vi "Pos_ImageIO.vi"(7 "Pos_ImageIO_commands":T2, 8 "Error In":errorcluster, 10 "Image File Path":path, 11 "ImageCluster IN":cluster{"Current Image":T1, "Saved Image":T1}) -> (0 "Error Out":errorcluster, 2 "Error!":bool, 3 "Saved Image OUT":T1)   [LabVIEW 2012]
uses:
  Pos_ImageIO_commands.ctl
  <vilib>/vision/Image Controls.llb/IMAQ Image.ctl
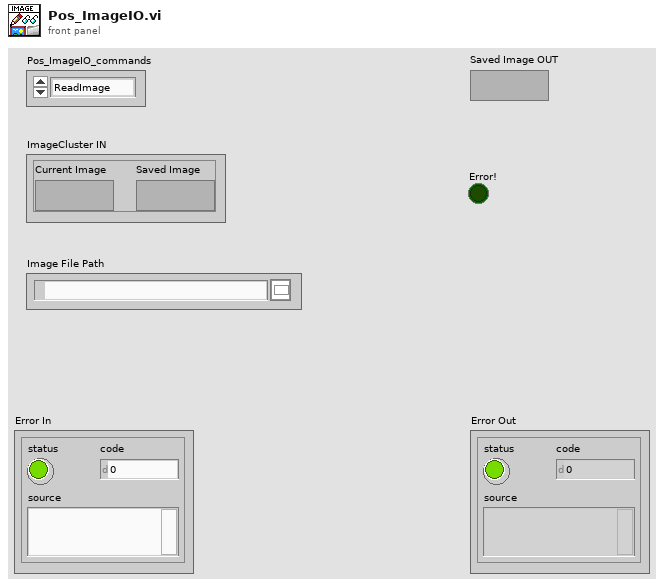
[diagram p1: front panel]
types:
  T1 = typedef "IMAQ Image.ctl" = refnum<image>
  T2 = typedef "Pos_ImageIO_commands.ctl" = enum16{"ReadImage", "WriteImage"}
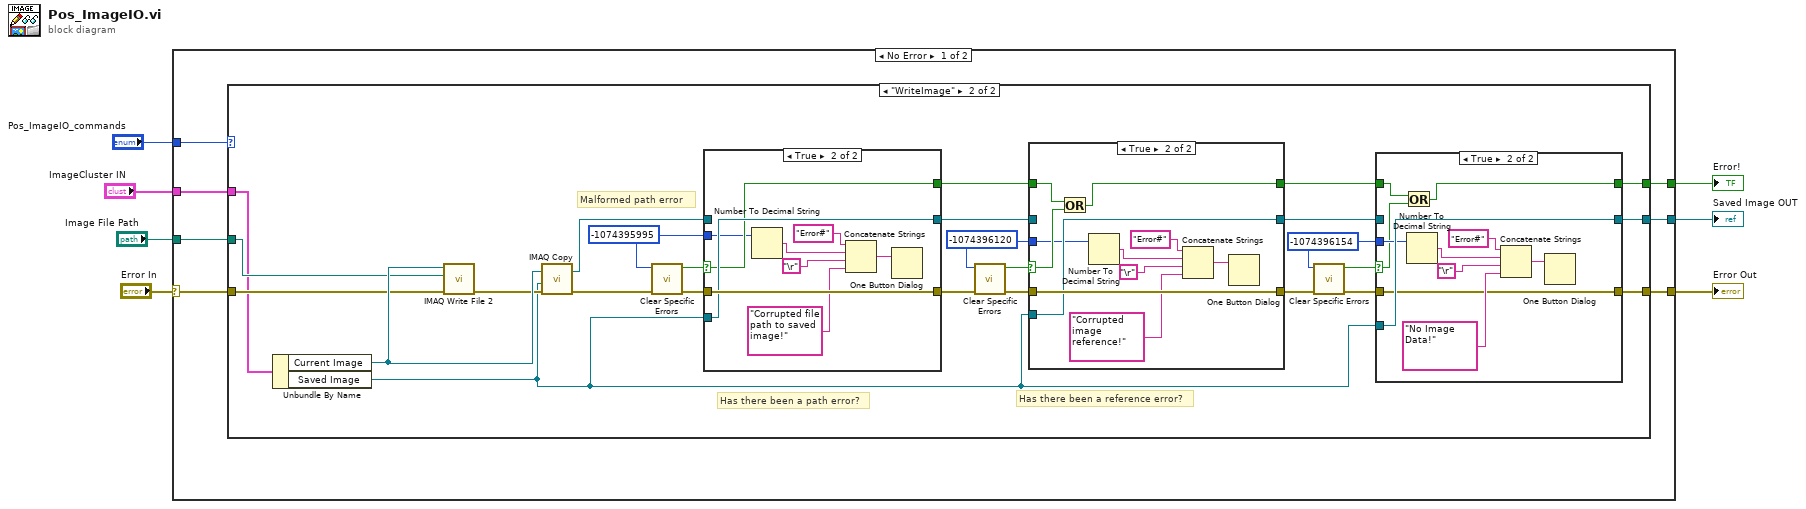
[diagram p0: block diagram]
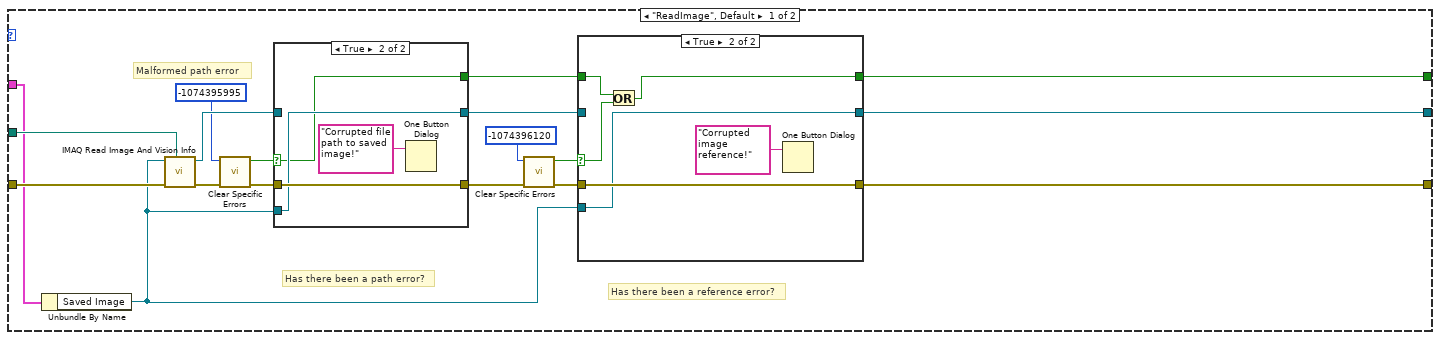
[diagram p2: hidden frame]
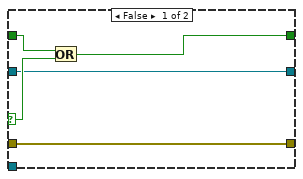
[diagram p3: hidden frame]
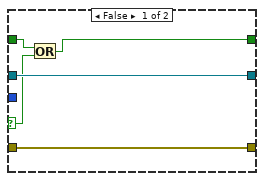
[diagram p5: hidden frame]
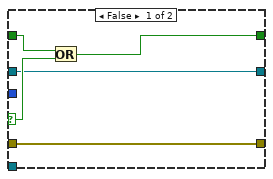
[diagram p6: hidden frame]
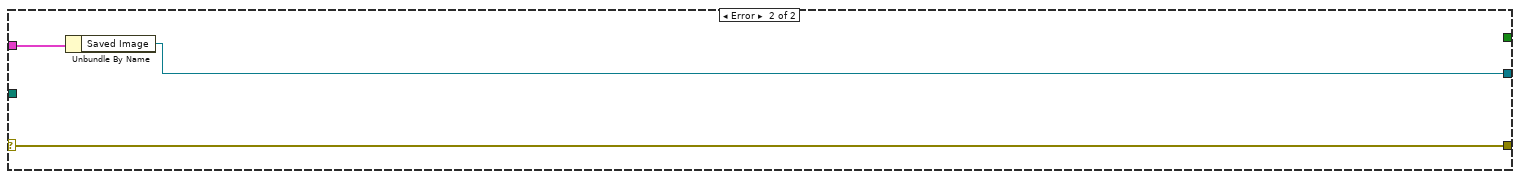
[diagram p8: hidden frame]
diagram:
  n1 = case shown="No Error" "Error In" {
    selector: "Error In" -> [w12 w119]
    tunnel: "Pos_ImageIO_commands" -> [w14 _]
    tunnel: "ImageCluster IN" -> [w13 w121]
    tunnel: "Image File Path" -> [w11 _]
    tunnel: [w10 w120] -> w4
    tunnel: [w9 w119] -> w3
    tunnel: [w8 _] -> w2
    frame No Error {
      n2 = case shown="\"WriteImage\"" w14 {
        tunnel: w13 -> [w25 w67]
        tunnel: w12 -> [w27 w73]
        tunnel: w11 -> [w26 w72]
        tunnel: [w17 w52] -> w10
        tunnel: [w21 w51] -> w9
        tunnel: [w18 w50] -> w8
        frame "ReadImage", Default {
          # "Has there been a path error?"
          # "Has there been a reference error?"
          # "Malformed path error"
          n3 = Unbundle By Name(w25) -> ("Saved Image"=w16:T1)
          n4 = call "IMAQ Read Image And Vision Info"("File Path"=w26, "error in (no error)"=w27, "Image"=w16) -> ("error out"=w31:errorcluster, "Image Out"=w32:T1)  [unwired: 6 in, 1 out]
          n5 = call "Clear Specific Errors.vi"("Error In"=w31, "Error number In"=-1074395995) -> ("Error Out"=w29:errorcluster, "Error Cleared?"=w30:bool)  [unwired: 8 in]
          n6 = case shown="True" w30 {
            selector: w30 -> [_ w46]
            tunnel: [w44 w48] -> w22
            tunnel: w32 -> [w45 _]
            tunnel: w29 -> [w44 w48]
            tunnel: [w45 w47] -> w20
            tunnel: w16 -> [_ w47]
            tunnel: [_ w46] -> w19
            frame False {
            }
            frame True {
              n7 = One Button Dialog(message="Corrupted file path to saved image!") -> ()  [unwired: 1 in, 1 out]
            }
          }
          n8 = call "Clear Specific Errors.vi"("Error In"=w22, "Error number In"=-1074396120) -> ("Error Out"=w24:errorcluster, "Error Cleared?"=w23:bool)  [unwired: 8 in]
          n9 = case shown="True" w23 {
            selector: w23 -> [w35 w42]
            tunnel: w24 -> [w37 w40]
            tunnel: w16 -> [_ w39]
            tunnel: w19 -> [w36 w43]
            tunnel: [w34 w41] -> w18
            tunnel: w20 -> [w33 _]
            tunnel: [w37 w40] -> w21
            tunnel: [w33 w39] -> w17
            frame False {
              n10 = Or(x=w36, y=w35) -> (x .or. y?=w34:bool)
            }
            frame True {
              n11 = Or(x=w43, y=w42) -> (x .or. y?=w41:bool)
              n12 = One Button Dialog(message="Corrupted image reference!") -> ()  [unwired: 1 in, 1 out]
            }
          }
        }
        frame "WriteImage" {
          w53 = -1074396154 ("Error number In")
          w54 = -1074396120 ("Error number In")
          w55 = -1074395995 ("Error number In")
          # "Has there been a reference error?"
          # "Has there been a path error?"
          # "Malformed path error"
          n13 = Unbundle By Name(w67) -> ("Current Image"=w75:T1, "Saved Image"=w59:T1)
          n14 = call-poly "IMAQ Write File 2"("error in (no error)"=w73, "File Path"=w72, "Image"=w75) -> ("error out"=w74:errorcluster)  [unwired: 7 in, 1 out]
          n15 = call "IMAQ Copy"("error in (no error)"=w74, "Image Dst"=w59, "Image Src"=w75) -> ("error out"=w69:errorcluster, "Image Dst Out"=w71:T1)  [unwired: 3 in]
          n16 = call "Clear Specific Errors.vi"("Error In"=w69, "Error number In"=w55) -> ("Error Out"=w70:errorcluster, "Error Cleared?"=w68:bool)  [unwired: 8 in]
          n17 = case shown="True" w68 {
            selector: w68 -> [_ w116]
            tunnel: [w108 w118] -> w66
            tunnel: w71 -> [w109 _]
            tunnel: w70 -> [w108 w118]
            tunnel: [w109 w117] -> w62
            tunnel: w59 -> [_ w117]
            tunnel: [_ w116] -> w63
            tunnel: w55 -> [_ w115]
            frame False {
            }
            frame True {
              n18 = Number To Decimal String(number=w115) -> (decimal integer string=w113:string)  [unwired: 1 in]
              n19 = Concatenate Strings("Error#", w113, "\r", "Corrupted file path to saved image!" ("message")) -> (w110:string)
              n20 = One Button Dialog(message=w110) -> ()  [unwired: 1 in, 1 out]
            }
          }
          n21 = call "Clear Specific Errors.vi"("Error In"=w66, "Error number In"=w54) -> ("Error Out"=w65:errorcluster, "Error Cleared?"=w64:bool)  [unwired: 8 in]
          n22 = case shown="True" w64 {
            selector: w64 -> [w94 w106]
            tunnel: w65 -> [w96 w104]
            tunnel: w59 -> [_ w103]
            tunnel: w63 -> [w95 w107]
            tunnel: [w93 w105] -> w60
            tunnel: w62 -> [w92 _]
            tunnel: [w96 w104] -> w58
            tunnel: [w92 w103] -> w61
            tunnel: w54 -> [_ w98]
            frame False {
              n23 = Or(x=w95, y=w94) -> (x .or. y?=w93:bool)
            }
            frame True {
              n24 = Or(x=w107, y=w106) -> (x .or. y?=w105:bool)
              n25 = Number To Decimal String(number=w98) -> (decimal integer string=w101:string)  [unwired: 1 in]
              n26 = Concatenate Strings("Error#", w101, "\r", "Corrupted image reference!" ("message")) -> (w99:string)
              n27 = One Button Dialog(message=w99) -> ()  [unwired: 1 in, 1 out]
            }
          }
          n28 = call "Clear Specific Errors.vi"("Error In"=w58, "Error number In"=w53) -> ("Error Out"=w57:errorcluster, "Error Cleared?"=w56:bool)  [unwired: 8 in]
          n29 = case shown="True" w56 {
            selector: w56 -> [w77 w82]
            tunnel: w61 -> [w79 _]
            tunnel: w60 -> [w78 w83]
            tunnel: w59 -> [_ w87]
            tunnel: w57 -> [w80 w84]
            tunnel: w53 -> [_ w86]
            tunnel: [w79 w87] -> w52
            tunnel: [w80 w84] -> w51
            tunnel: [w76 w81] -> w50
            frame False {
              n30 = Or(x=w78, y=w77) -> (x .or. y?=w76:bool)
            }
            frame True {
              n31 = Or(x=w83, y=w82) -> (x .or. y?=w81:bool)
              n32 = Number To Decimal String(number=w86) -> (decimal integer string=w89:string)  [unwired: 1 in]
              n33 = Concatenate Strings("Error#", w89, "\r", "No Image Data!" ("message")) -> (w91:string)
              n34 = One Button Dialog(message=w91) -> ()  [unwired: 1 in, 1 out]
            }
          }
        }
      }
    }
    frame Error {
      n35 = Unbundle By Name(w121) -> ("Saved Image"=w120:T1)
    }
  }
  "Error Out" <- w3
  "Saved Image OUT" <- w4
  "Error!" <- w2
